vi "interpolate_to_nearest.vi"(8 "start index (0)":i32, 9 "round mode (nerest)":enum16{"nearest", "floor", "ceil"}(ring), 10 "value":dbl, 11 "array":dbl[](array[numeric])) -> (2 "nearest index":i32, 3 "nearest value":dbl)   [LabVIEW 2015]
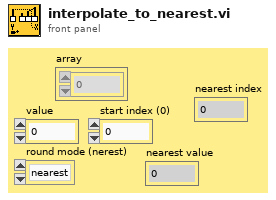
[diagram p1: front panel]
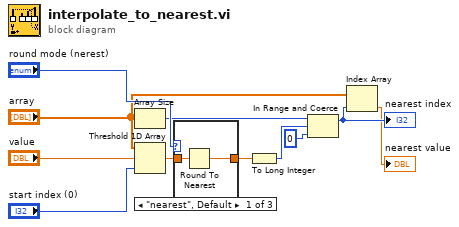
[diagram p0: block diagram]
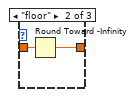
[diagram p2: hidden frame]
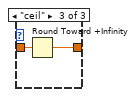
[diagram p3: hidden frame]
diagram:
  n1 = Array Size(array="array") -> (size(s)=w4:i32)
  n2 = Threshold 1D Array(1:"start index (0)", 2:"value", 3:"array") -> (0:w11:dbl)
  n3 = case shown="\"nearest\", Default" "round mode (nerest)" {
    tunnel: w11 -> [w13 w15 w17]
    tunnel: [w12 w14 w16] -> w10
    frame "nearest", Default {
      n4 = Round To Nearest(number=w13) -> (nearest integer value=w12:dbl)
    }
    frame "floor" {
      n5 = Round Toward -Infinity(1:w15) -> (0:w14:dbl)
    }
    frame "ceil" {
      n6 = Round Toward +Infinity(x=w17) -> (ceil(x): smallest int >= x=w16:dbl)
    }
  }
  n7 = To Long Integer(number=w10) -> (32bit integer=w6:i32)
  n8 = In Range and Coerce(upper limit=w4, x=w6, lower limit=0) -> (coerced(x)=w2:i32)  [unwired: 1 out]
  "nearest index" <- w2
  n9 = Index Array(array="array", index=w2) -> (element=→"nearest value":dbl)
